vi "Flush Log File.vi"(8 "error in (no error)":errorcluster, 11 "Log File in":refnum<class "Log File.lvclass">) -> (0 "error out":errorcluster, 3 "Log File out":refnum<class "Log File.lvclass">)   [LabVIEW 2012, in "Waveform Data Logger Engine.lvlib" / "Log File.lvclass"]
uses:
  Log File.lvclass
  Log File.lvclass/Log File.ctl
  TDMS Log File/TDMS Log File.lvclass
  Text Log File/Text Log File.lvclass
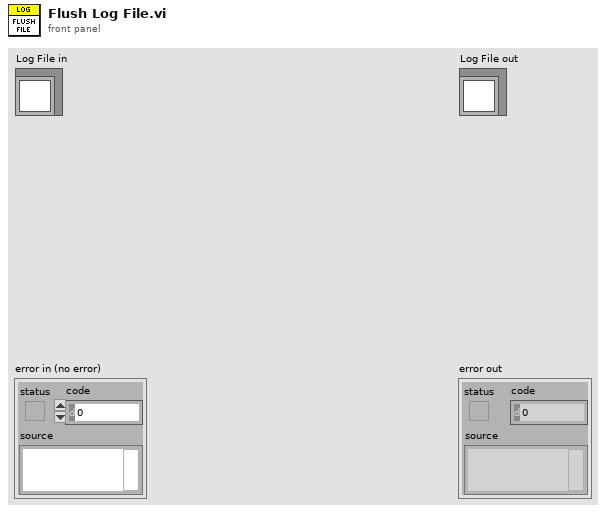
[diagram p1: front panel]
types:
  T1 = typedef "Waveform Data Logger Engine.lvlib/Log File.lvclass/Log File Type.ctl" = enum16{"Default", "TDMS", "Text"}
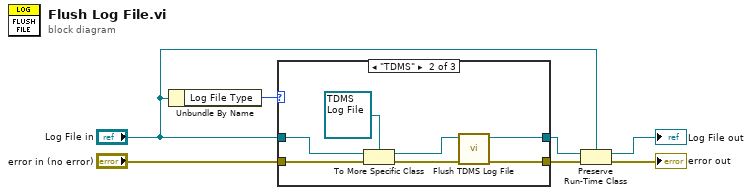
[diagram p0: block diagram]
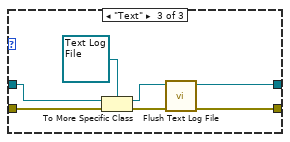
[diagram p3: hidden frame]
diagram:
  n1 = Unbundle By Name("Log File in") -> ("Log File Type"=w7:T1)
  n2 = case shown="\"TDMS\"" w7 {
    tunnel: "error in (no error)" -> [w9 w16 w22]
    tunnel: [w9 w11 w23] -> w5
    tunnel: "Log File in" -> [w8 w15 w20]
    tunnel: [w8 w10 w17] -> w3
    frame "Default", Default {
    }
    frame "TDMS" {
      n3 = To More Specific Class(target class=refnum<class "TDMS Log File.lvclass"> refnum ("TDMS Log File.lvclass"), reference=w15, error in=w16) -> (specific class reference=w13:refnum<class "TDMS Log File.lvclass">, error out=w12:errorcluster)
      n4 = call "Flush TDMS Log File.vi"("error in (no error)"=w12, "TDMS Log File in"=w13) -> ("error out"=w11:errorcluster, "TDMS Log File out"=w10:refnum<class "TDMS Log File.lvclass">)  [unwired: 8 in]
    }
    frame "Text" {
      n5 = To More Specific Class(target class=refnum<class "Text Log File.lvclass"> refnum ("Text Log File.lvclass"), reference=w20, error in=w22) -> (specific class reference=w18:refnum<class "Text Log File.lvclass">, error out=w21:errorcluster)
      n6 = call "Flush Text Log File.vi"("error in (no error)"=w21, "Text Log File in"=w18) -> ("error out"=w23:errorcluster, "Text Log File out"=w17:refnum<class "Text Log File.lvclass">)  [unwired: 8 in]
    }
  }
  n7 = Preserve Run-Time Class(object in=w3, error in=w5, 2:"Log File in") -> (object out=→"Log File out":refnum<class "Log File.lvclass">, error out=→"error out":errorcluster)
